vi "register_hmi_references.vi"(8 "error in (no error)":errorcluster, 11 "hmi_references":T1) -> (0 "error out":errorcluster, 3 "external":T2)   [LabVIEW 2015, in "functional.lvlib"]
uses:
  functional.lvlib
  _controls/event_registration_external.ctl
  public/_controls/hmi_references.ctl
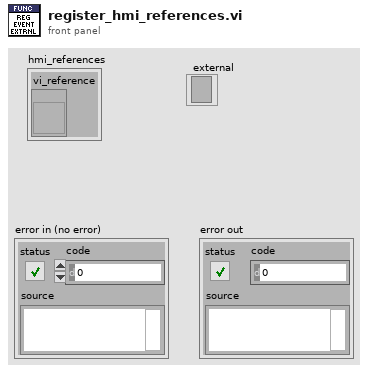
[diagram p1: front panel]
types:
  T1 = typedef "functional.lvlib/hmi_references.ctl" = cluster{"vi_reference":refnum<vi>}
  T2 = typedef "functional.lvlib/event_registration_external.ctl" = refnum<event-registration>
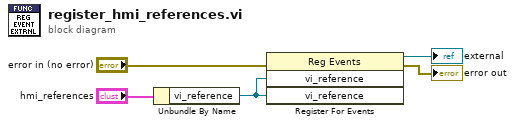
[diagram p0: block diagram]
diagram:
  n1 = Unbundle By Name("hmi_references") -> ("vi_reference"=w2:refnum<vi>)
  n2 = register-events(error in="error in (no error)", w2, w2) -> (reference out=→"external":refnum<event-registration>, error out=→"error out":errorcluster)  [unwired: 1 in]
